vi "b2b.vi"   [LabVIEW 2016, in "Moving Motor.lvrbt"]
uses:
  Moving Motor.lvrbt
  <vilib>/NXT/Hardware/Plugins/Tetrix DC Motor/TetrixDCMotorAddress.ctl
  <vilib>/NXT/Block Support/NXT_InputPort.ctl
  <vilib>/NXT/NXTIO Xnodes/NXTIONodeSubVIs/TETRIX IO Move DC Motors.vi
  <vilib>/NXT/NXTIO Xnodes/NXTIONodeSubVIs/TETRIX IO Stop DC Motors.vi
  <vilib>/NXT/Dual Mode Library/Sensors/EV3_Color_Color.vi
  <vilib>/NXT/Subs/LVHSConnector.ctl
  <vilib>/NXT/NXTIO Xnodes/AddressXNode/NXTIOAddress.xnode
  <vilib>/NXT/NXTIO Xnodes/NXTIOXNode/NXTIO.xnode
  <vilib>/NXT/LegoClasses/BrickReference/BrickReference.lvclass
types:
  T1 = typedef "TetrixDCMotorAddress.ctl" = i32
  T2 = typedef "LVHSConnector.ctl" = refnum<class "BrickReference.lvclass">
  T3 = typedef "NXT_InputPort.ctl" = u32
  T4 = typedef "ColorSensorColors.ctl" = enum16{"No Color", "Black", "Blue", "Green", "Yellow", "Red", "White", "Brown"}
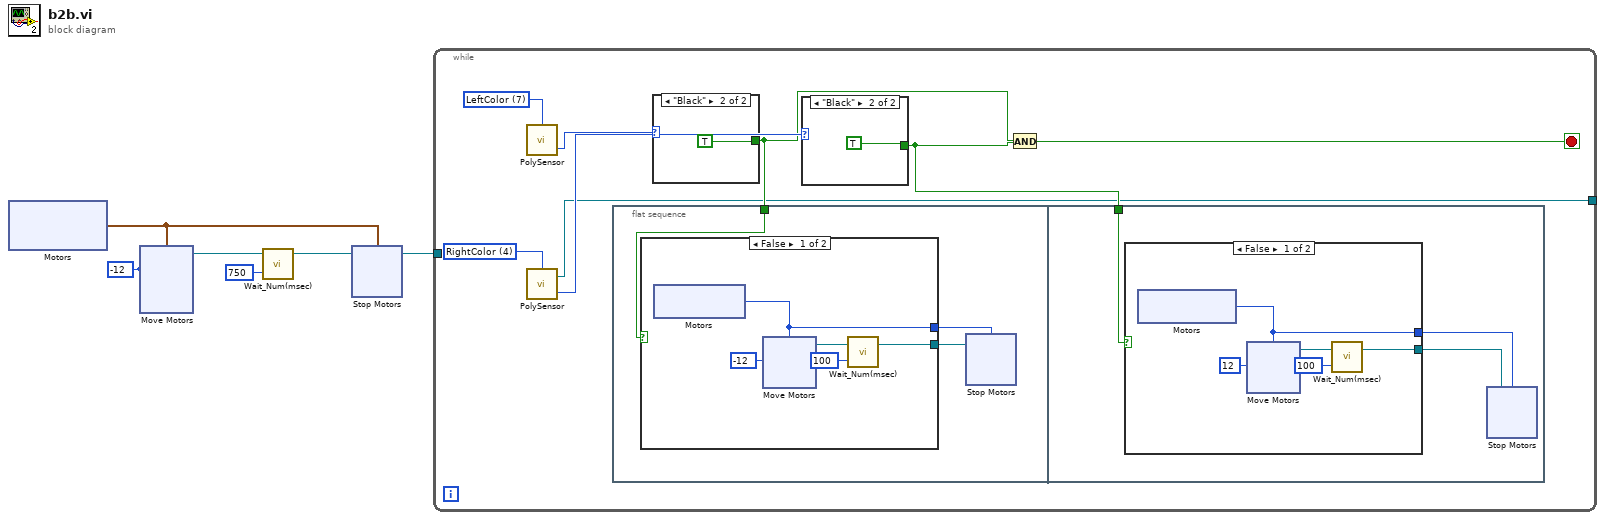
[diagram p0: block diagram]
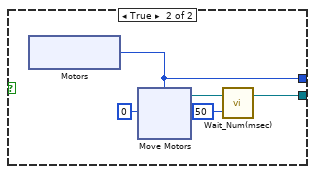
[diagram p2: hidden frame]
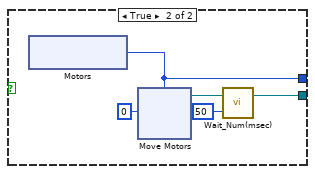
[diagram p3: hidden frame]
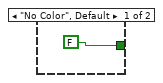
[diagram p4: hidden frame]
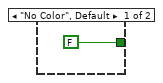
[diagram p5: hidden frame]
diagram:
  w6 = i8 -12 ("Power/Speed 1")
  n1 = xnode "Motors"() -> ("Motor"=w2:cluster{"TetrixDCMotor":T1, "TetrixDCMotor":T1})
  n2 = xnode "Move Motors"("Power/Speed 2"=w6, "Power/Speed 1"=w6, "Motors"=w2) -> ("NXT/EV3"=w5:T2)  [unwired: 1 in]
  n3 = call <vilib>:"Wait_Num(msec).vi"("Time (100 msec)"=u32 750, "NXT/EV3"=w5) -> ("NXT/EV3"=w3:T2)  [unwired: 2 in]
  n4 = xnode "Stop Motors"("Motors"=w2, "NXT/EV3"=w3) -> ("NXT/EV3"=w1:T2)
  n5 = while {
    tunnel: w1 -> [_]
    tunnel: [w7] -> _
    stop <- w10 stop-if-true
    w13 = T3 4 items=["Port 1", "Port 2", "Port 3", "Port 4", "RightColor"] ("Port (Port 1)")
    w14 = T3 7 items=["Port 1"=0, "Port 2"=1, "Port 3"=2, "Port 4"=3, "LeftColor"=7] ("Port (Port 1)")
    n6 = call-poly <vilib>:"PolySensor.vi"("Port (Port 1)"=w14) -> ("Detected Color"=w12:T4)  [unwired: 2 in, 1 out]
    n7 = call-poly <vilib>:"PolySensor.vi"("Port (Port 1)"=w13) -> ("Detected Color"=w11:T4, "NXT/EV3"=w7:T2)  [unwired: 2 in]
    n8 = flat-sequence {
      tunnel: w9 -> [w17]
      tunnel: w8 -> [w49]
      frame #0 {
        n9 = case shown="False" w17 {
          tunnel: [w24 w37] -> w16
          tunnel: [w23 w36] -> w15
          frame False {
            n10 = xnode "Motors"() -> ("Motor"=w23:T1)
            n11 = xnode "Move Motors"("Power/Speed 1"=i8 -12, "Motors"=w23) -> ("NXT/EV3"=w27:T2)  [unwired: 1 in]
            n12 = call <vilib>:"Wait_Num(msec).vi"("Time (100 msec)"=u32 100, "NXT/EV3"=w27) -> ("NXT/EV3"=w24:T2)  [unwired: 2 in]
          }
          frame True {
            n13 = xnode "Motors"() -> ("Motor"=w36:T1)
            n14 = xnode "Move Motors"("Power/Speed 1"=i8 0, "Motors"=w36) -> ("NXT/EV3"=w38:T2)  [unwired: 1 in]
            n15 = call <vilib>:"Wait_Num(msec).vi"("Time (100 msec)"=u32 50, "NXT/EV3"=w38) -> ("NXT/EV3"=w37:T2)  [unwired: 2 in]
          }
        }
        n16 = xnode "Stop Motors"("Motors"=w15, "NXT/EV3"=w16) -> ()  [unwired: 1 out]
      }
      frame #1 {
        n17 = case shown="False" w49 {
          tunnel: [w58 w71] -> w51
          tunnel: [w57 w70] -> w50
          frame False {
            n18 = xnode "Motors"() -> ("Motor"=w57:T1)
            n19 = xnode "Move Motors"("Power/Speed 1"=i8 12, "Motors"=w57) -> ("NXT/EV3"=w61:T2)  [unwired: 1 in]
            n20 = call <vilib>:"Wait_Num(msec).vi"("Time (100 msec)"=u32 100, "NXT/EV3"=w61) -> ("NXT/EV3"=w58:T2)  [unwired: 2 in]
          }
          frame True {
            n21 = xnode "Motors"() -> ("Motor"=w70:T1)
            n22 = xnode "Move Motors"("Power/Speed 1"=i8 0, "Motors"=w70) -> ("NXT/EV3"=w72:T2)  [unwired: 1 in]
            n23 = call <vilib>:"Wait_Num(msec).vi"("Time (100 msec)"=u32 50, "NXT/EV3"=w72) -> ("NXT/EV3"=w71:T2)  [unwired: 2 in]
          }
        }
        n24 = xnode "Stop Motors"("Motors"=w50, "NXT/EV3"=w51) -> ()  [unwired: 1 out]
      }
    }
    n25 = case shown="\"Black\"" w12 {
      tunnel: [FALSE TRUE] -> w9
      frame "No Color", Default {
      }
      frame "Black" {
      }
    }
    n26 = case shown="\"Black\"" w11 {
      tunnel: [FALSE TRUE] -> w8
      frame "No Color", Default {
      }
      frame "Black" {
      }
    }
    n27 = And(x=w9, y=w8) -> (x .and. y?=w10:bool)
  }
